vi "Main.vi"() -> ()   [LabVIEW 2019]
doc: "管道泄漏检测系统主程序"
uses:
  SSH Library/Connection Info..cluster.ctl
  SSH Library/Password..cluster.ctl
  References/PythonVersionsEnum.ctl
  <vilib>/Utility/miscctls.llb/LVForegroundBackgroundColorsTypeDef.ctl
  SSH Library/connect_password.vi
  SSH Library/connect_key.vi
  SFTP Library/connect_password.vi
  SFTP Library/connect_key.vi
  <vilib>/Utility/file.llb/Read Delimited Spreadsheet (DBL).vi
  SSH Library/LabSSH.lvlib
  SFTP Library/LabSFTP.lvlib
panel:
  out "泄漏点位置":sgl
  in  "管长":i32=100
  in  "时间间隔":string="10"
  in  "重复次数":string="3"
  in  "开始时间":string="140300"
  in  "开始日期":string="20200810"
  in  "增益":string="1"
  in  "采样率":string="6"
  out "混合信号图":T1(graph)
  in  "关闭":bool
  in  "运行":bool
  in  "选项卡控件":enum32{"系统模型", "设备参数设置", "输出显示"}(tab)=enum."设备参数设置"
  out "布尔 10":bool
  out "布尔 9":bool
  out "Multi-Segment Pipe 2":bool(c317)
  out "布尔 8":bool
  out "布尔 7":bool
  out "布尔 6":bool
  out "布尔 5":bool
  out "布尔 4":bool
  out "布尔 3":bool
  out "布尔 2":bool
  out "Multi-Segment Pipe":bool(c317)
  in  "1号设备连接信息":T2={"IP地址"="192.168.137.140", "用户名"="pi", "端口 (22)"=22}
  in  "Password 1":T3={"密码"="zjl"}
  out "isSshConnected":bool
  out "SSH响应":string
  in  "Connection Type":enum16{"Password", "Private Key"}(ring)
  in  "Expected Response":string="raspberrypi："
  in  "Password 2":T3={"密码"="raspberry"}
  in  "2号设备连接信息":T2={"IP地址"="192.168.137.224", "用户名"="pi", "端口 (22)"=22}
  in  "Password 3":T3={"密码"="raspberry"}
  in  "3号设备连接信息":T2={"IP地址"="192.168.137.224", "用户名"="pi", "端口 (22)"=22}
  out "SFTP响应":string
  out "isSftpConnected":bool
  out "Output":string
  out "运行状态":bool
  out "诊断结论":string
  in  "采样点数":string="2000"
  in  "通道号":string="0"
  out "进度条":dbl(slide) scale=0.0..1.0
  out "开始时间":dbl=18702.3337437 caption="相对秒钟" format="%_19f"
  in  "采集命令":string="cd /home/pi/leakad\nsudo ./pipedaq  0  2000  5  1"
  out "日期字符串":string="2020/5/27"
  out "时间字符串":string="13:45:51"
  # "管道泄漏监测系统"
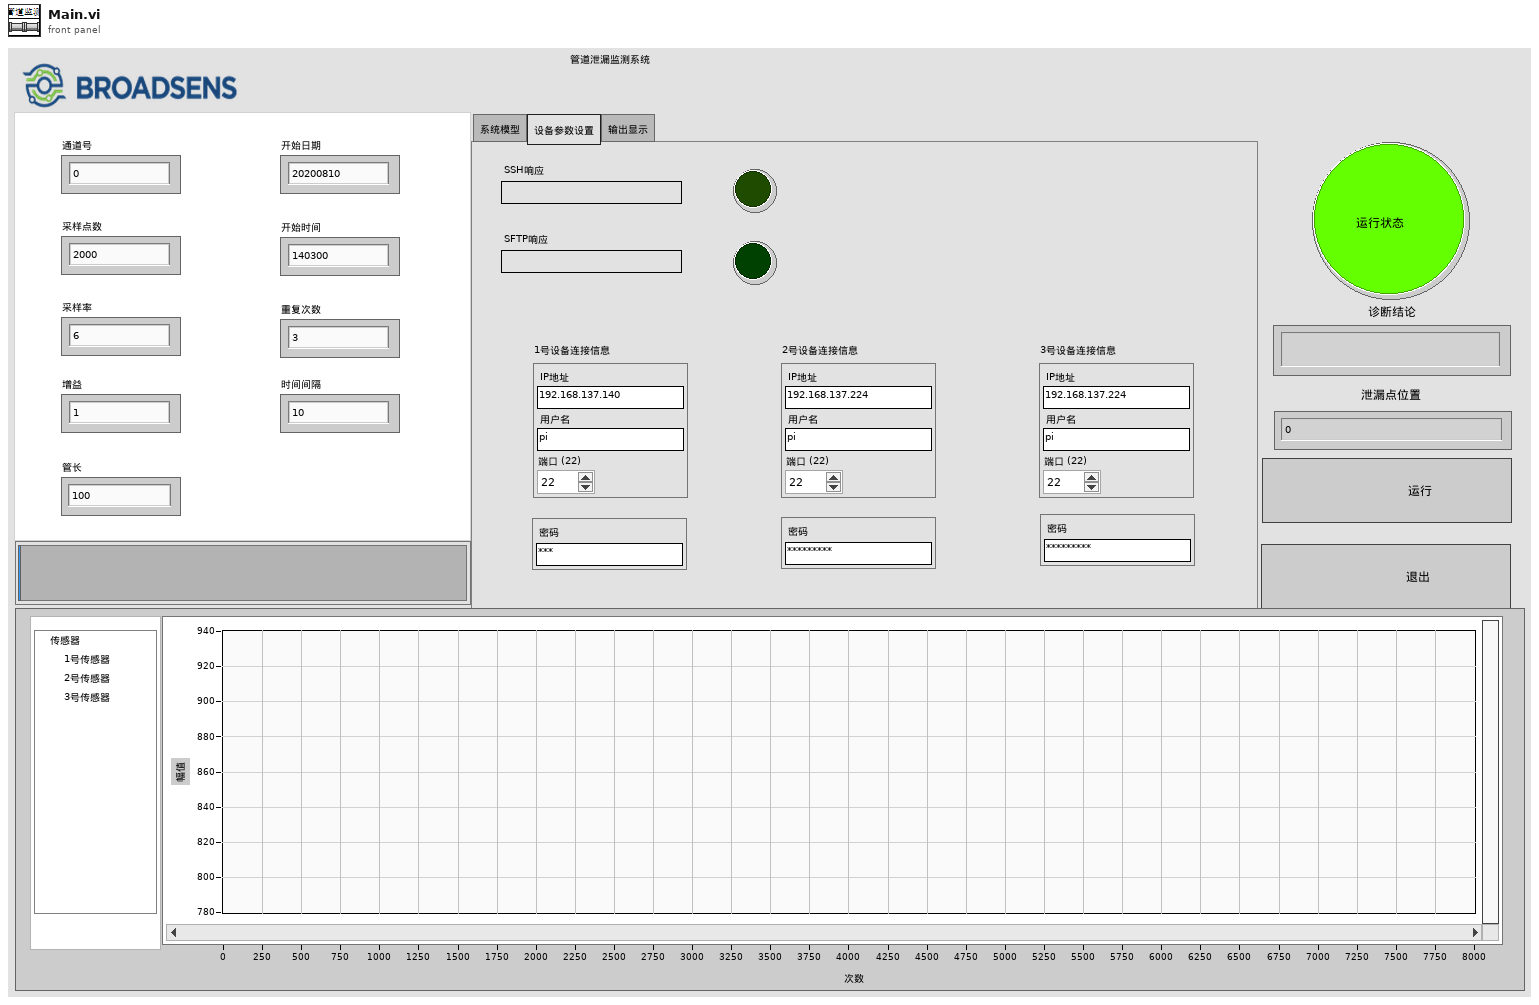
[diagram p1: front panel]
types:
  T1 = cluster{"first row":dbl[], "first row":dbl[], "first row":dbl[]}
  T2 = typedef "LabSSH.lvlib/Connection Info..cluster.ctl" = cluster{"IP地址":string, "用户名":string, "端口 (22)":i32}
  T3 = typedef "LabSSH.lvlib/Password..cluster.ctl" = cluster{"密码":string}
  T4 = enum32{"Invalid", "Standard", "Closed", "Hidden", "Minimized", "Maximized"}
  T5 = enum32{"invalid app kind", "Development System", "Run Time System", "Student Edition", "Embedded LabVIEW", "Evaluation", "Custom"}
  T6 = typedef "PythonVersionsEnum.ctl" = enum16{"2.7", "3.6"}
  T7 = typedef "LVForegroundBackgroundColorsTypeDef.ctl" = cluster{"Foreground Color":u32, "Background Color":u32}
  T8 = cluster{"Core":cluster{"Current VI Reference":refnum<vi>, "Close Panel on Exit?":bool}, "Your Boolean data":bool, "Your string data":string}
  T9 = cluster{"Current VI Reference":refnum<vi>, "Close Panel on Exit?":bool}
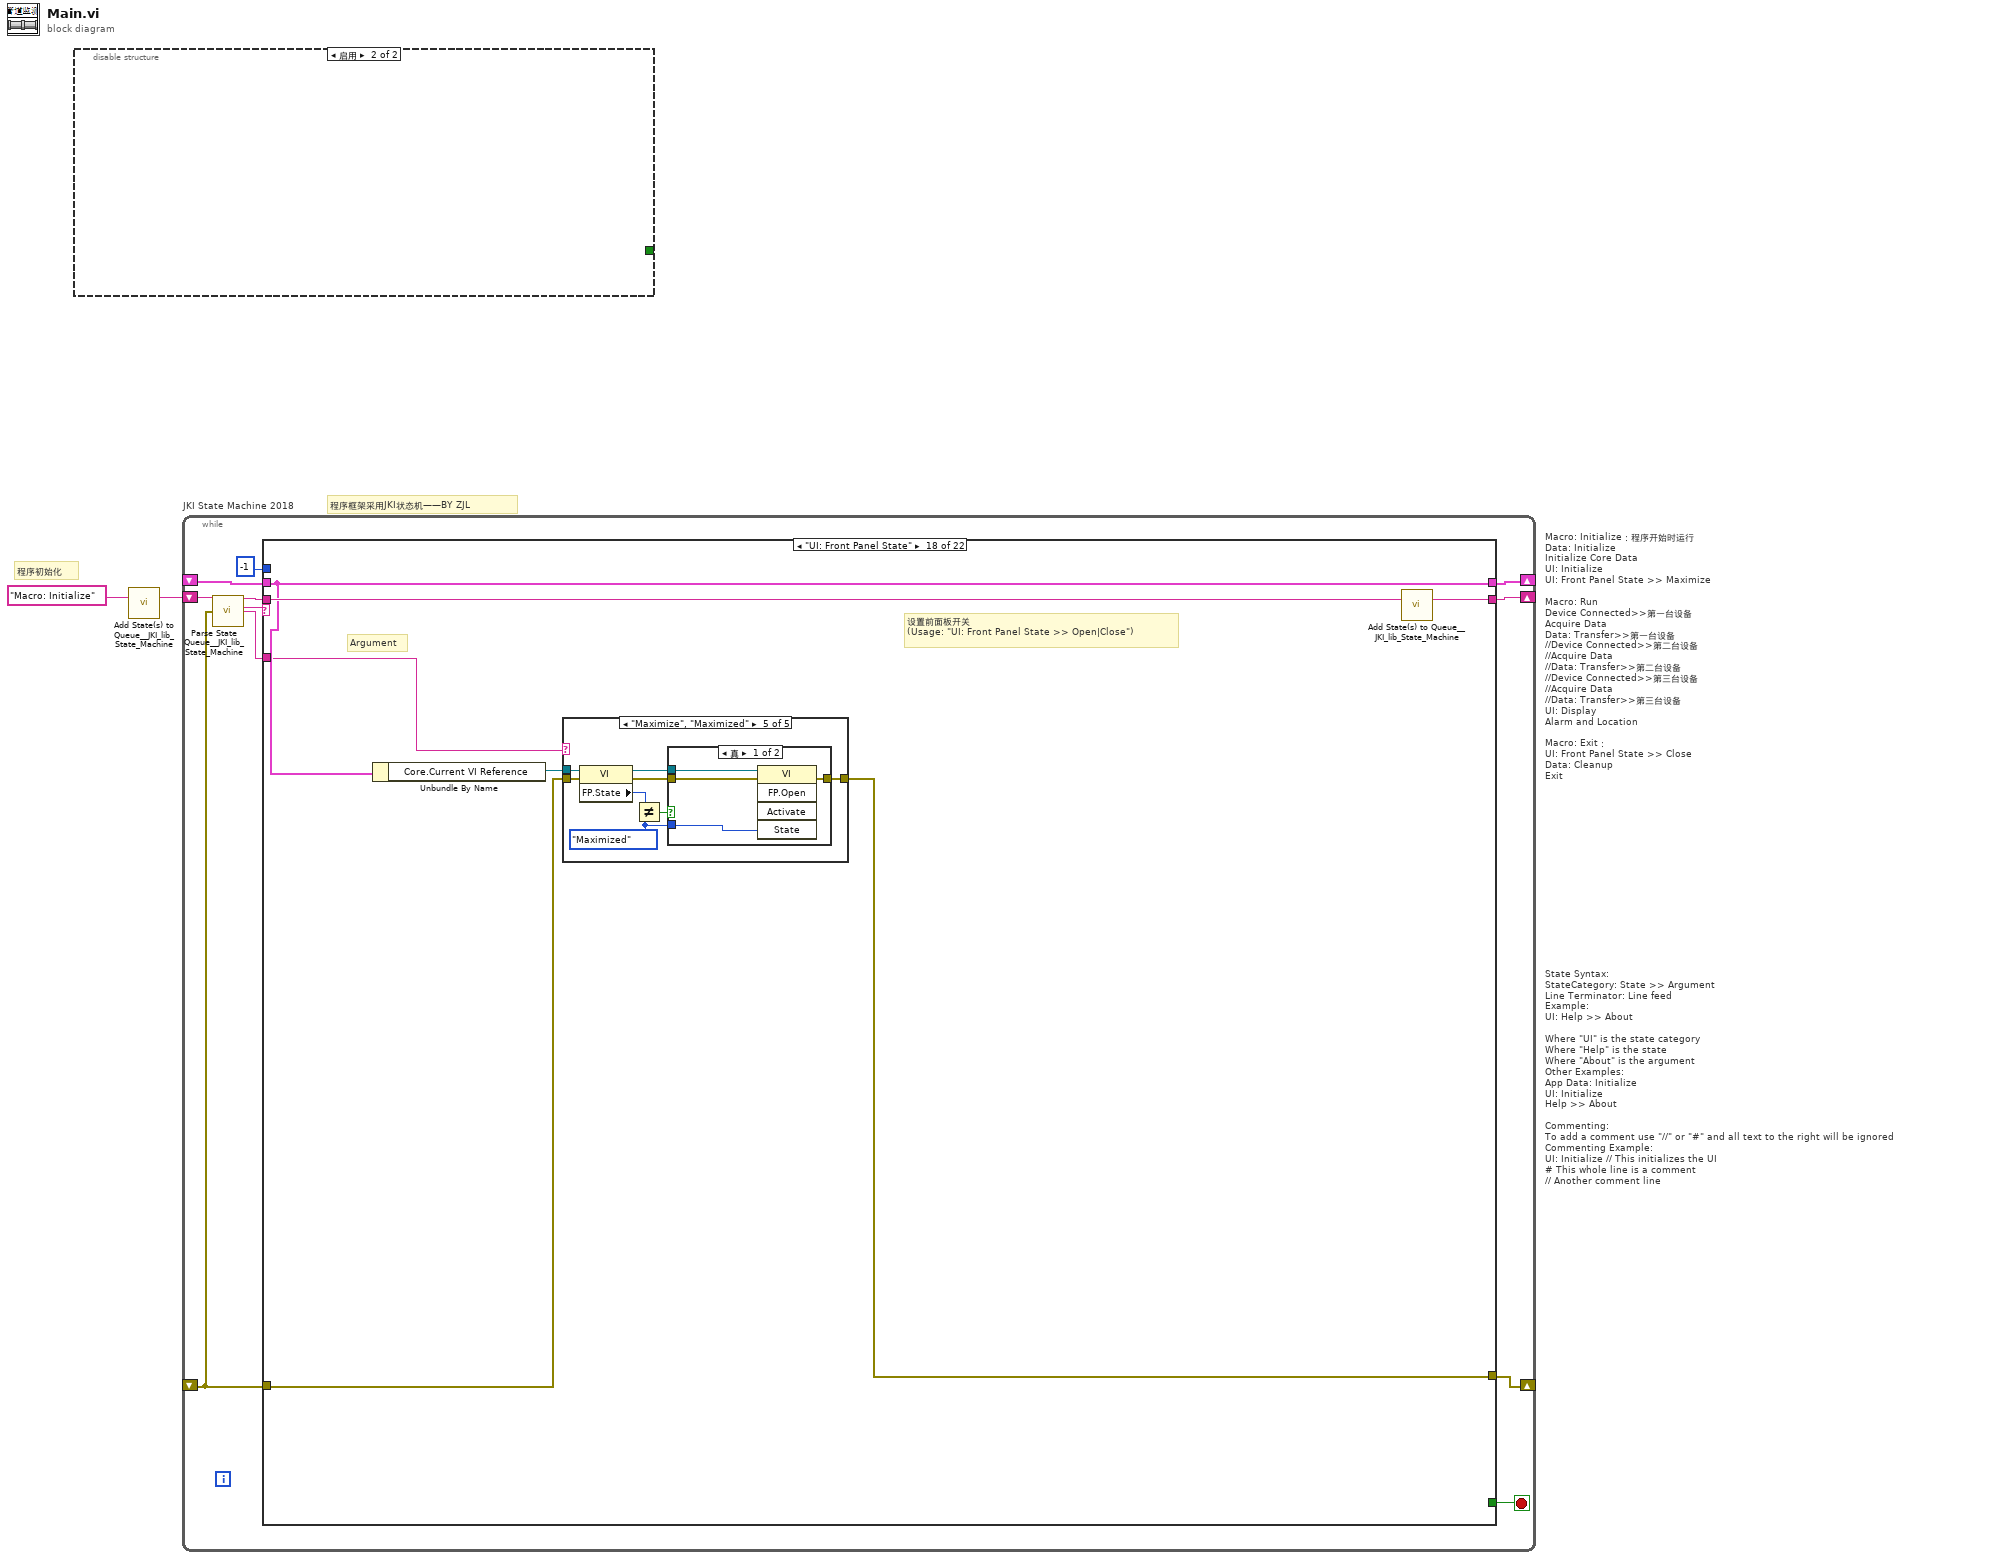
[diagram p0: block diagram]
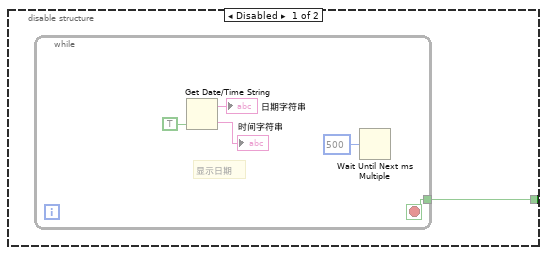
[diagram p2: hidden frame]
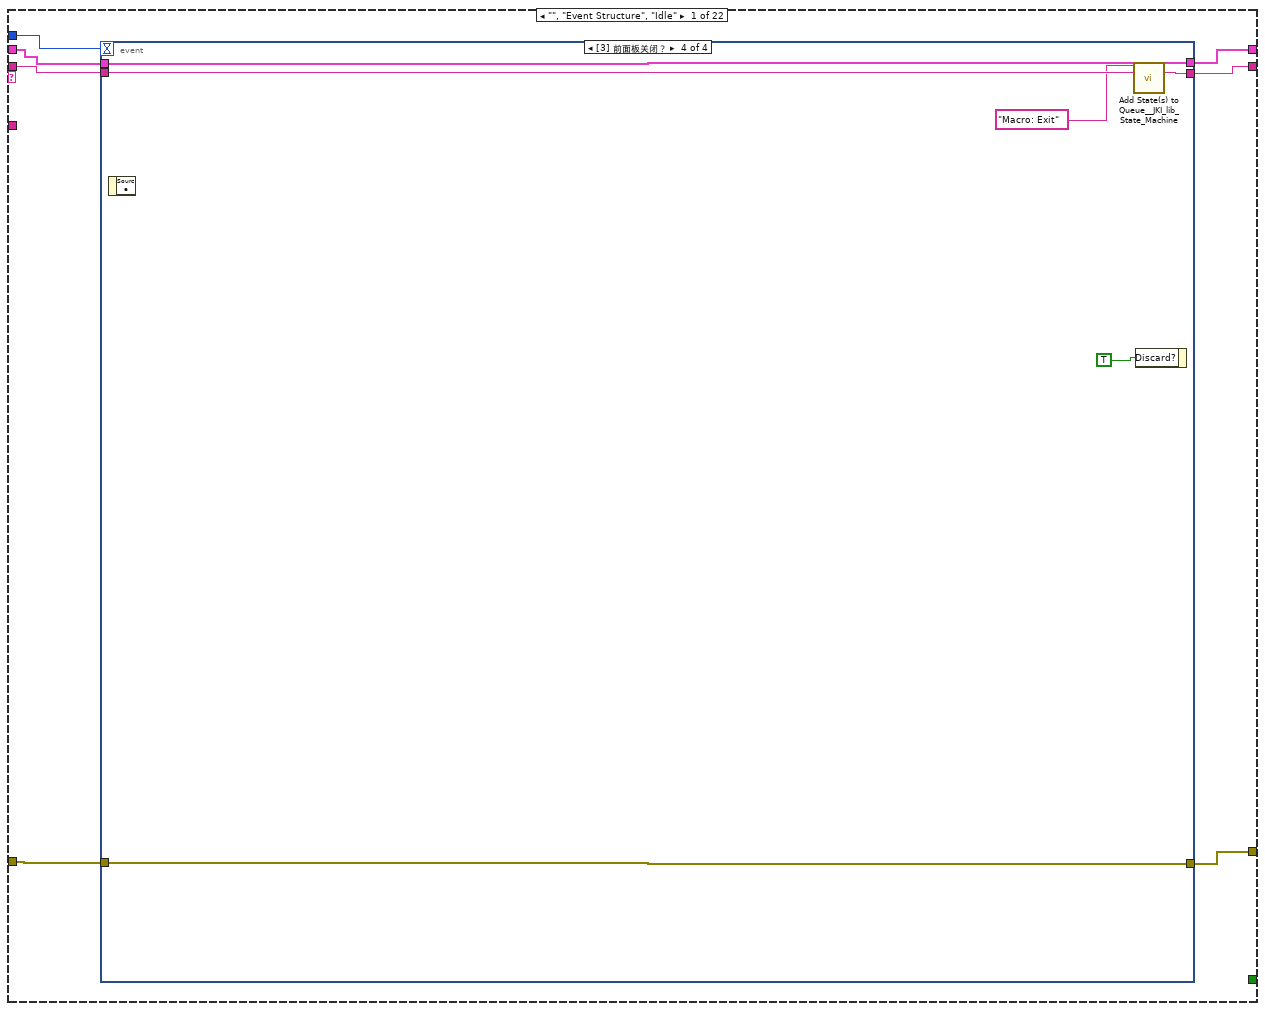
[diagram p3: hidden frame]
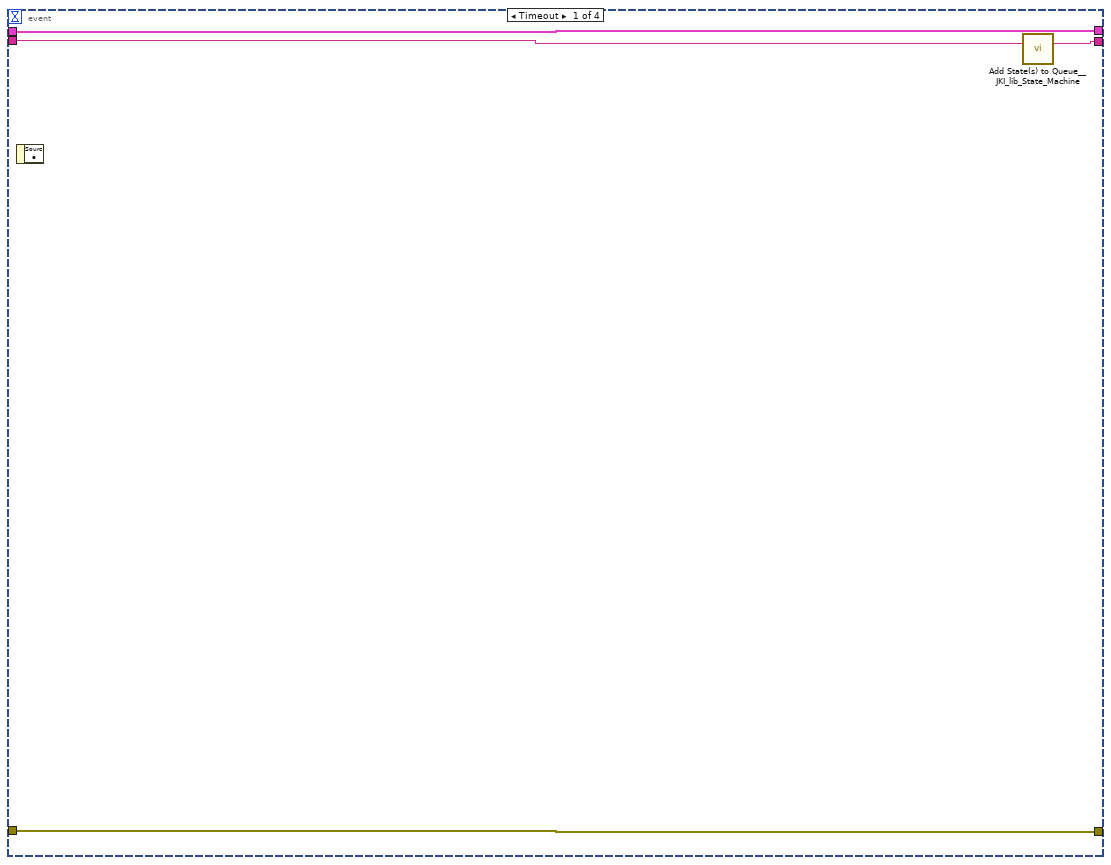
[diagram p4: hidden frame]
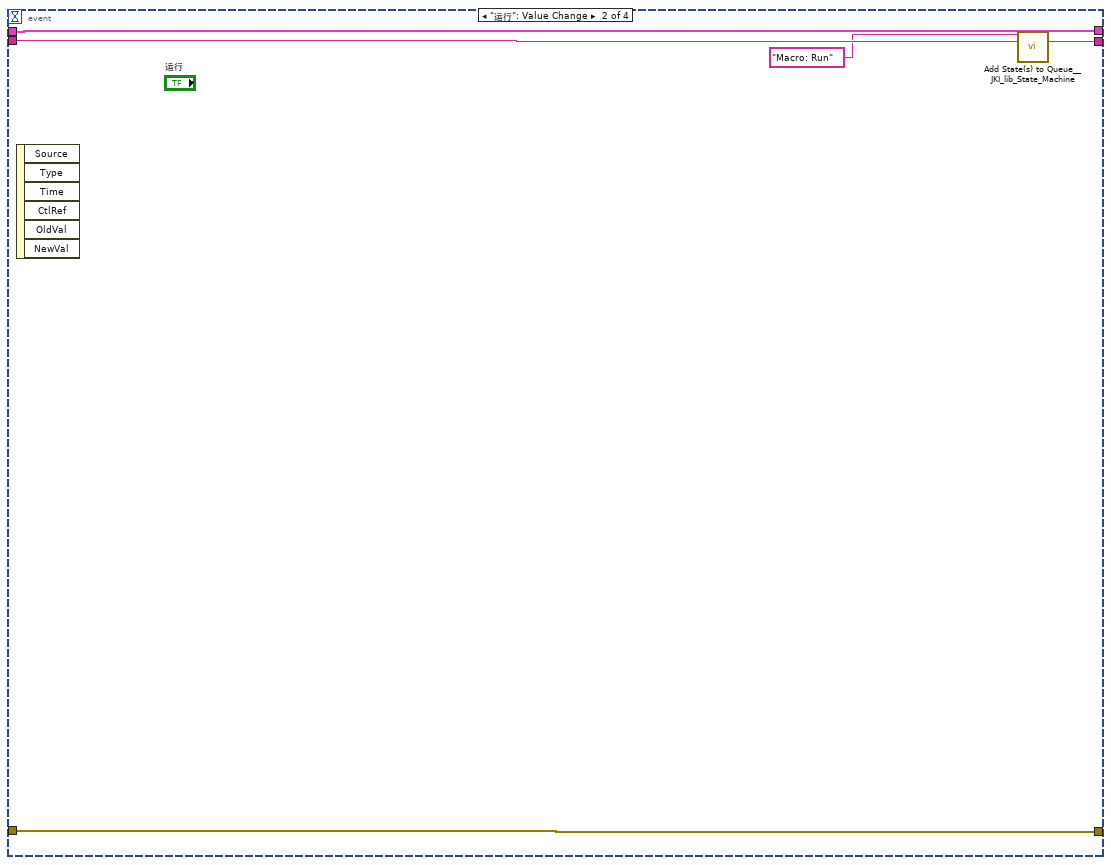
[diagram p5: hidden frame]
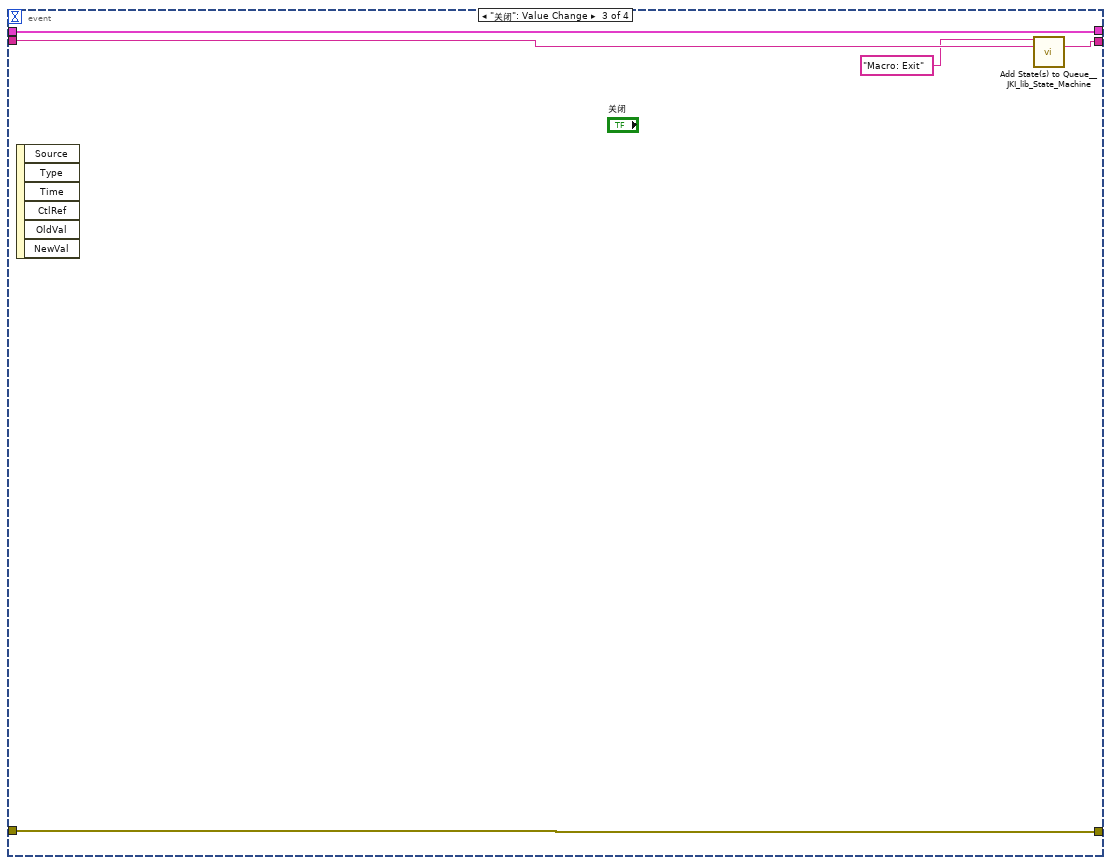
[diagram p6: hidden frame]
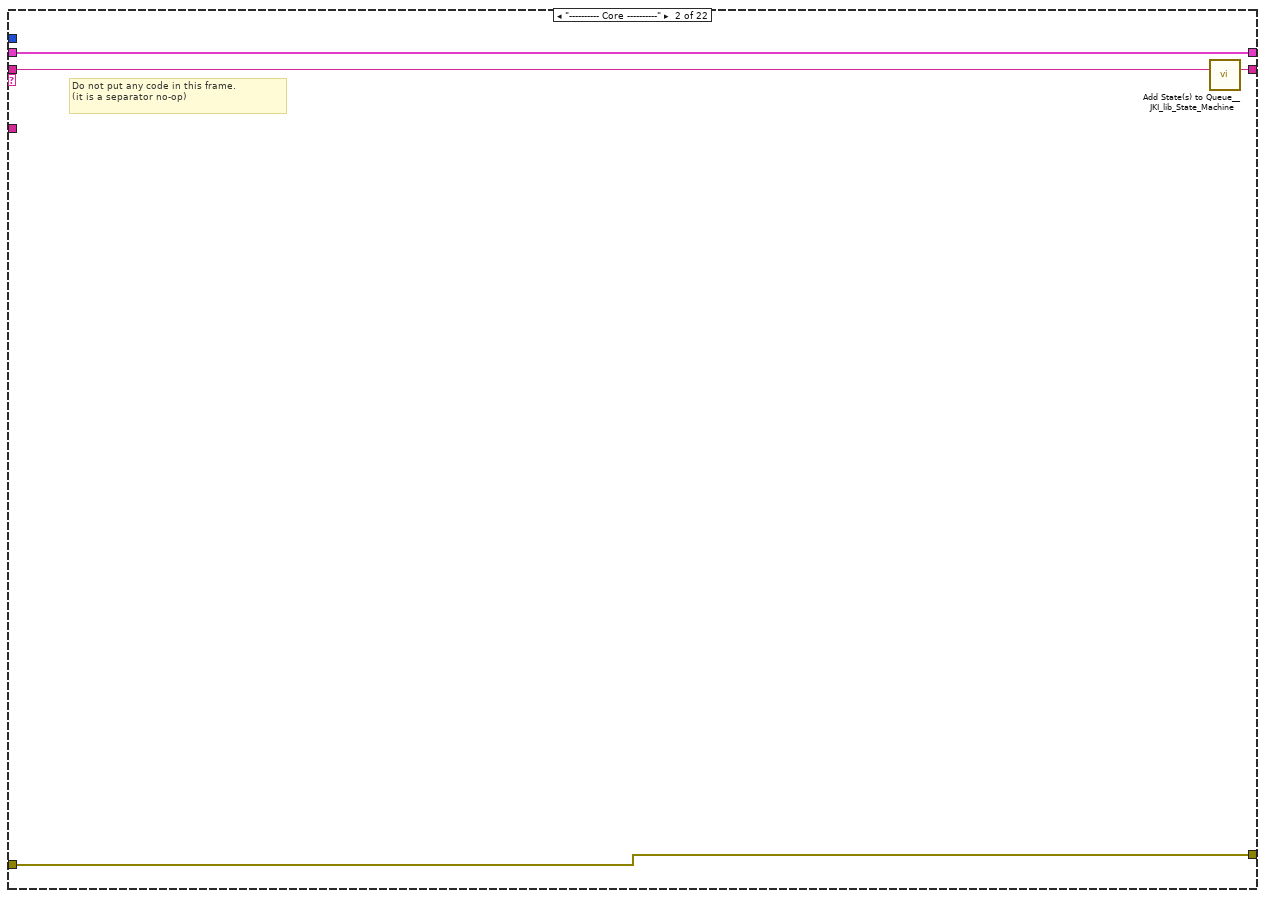
[diagram p7: hidden frame]
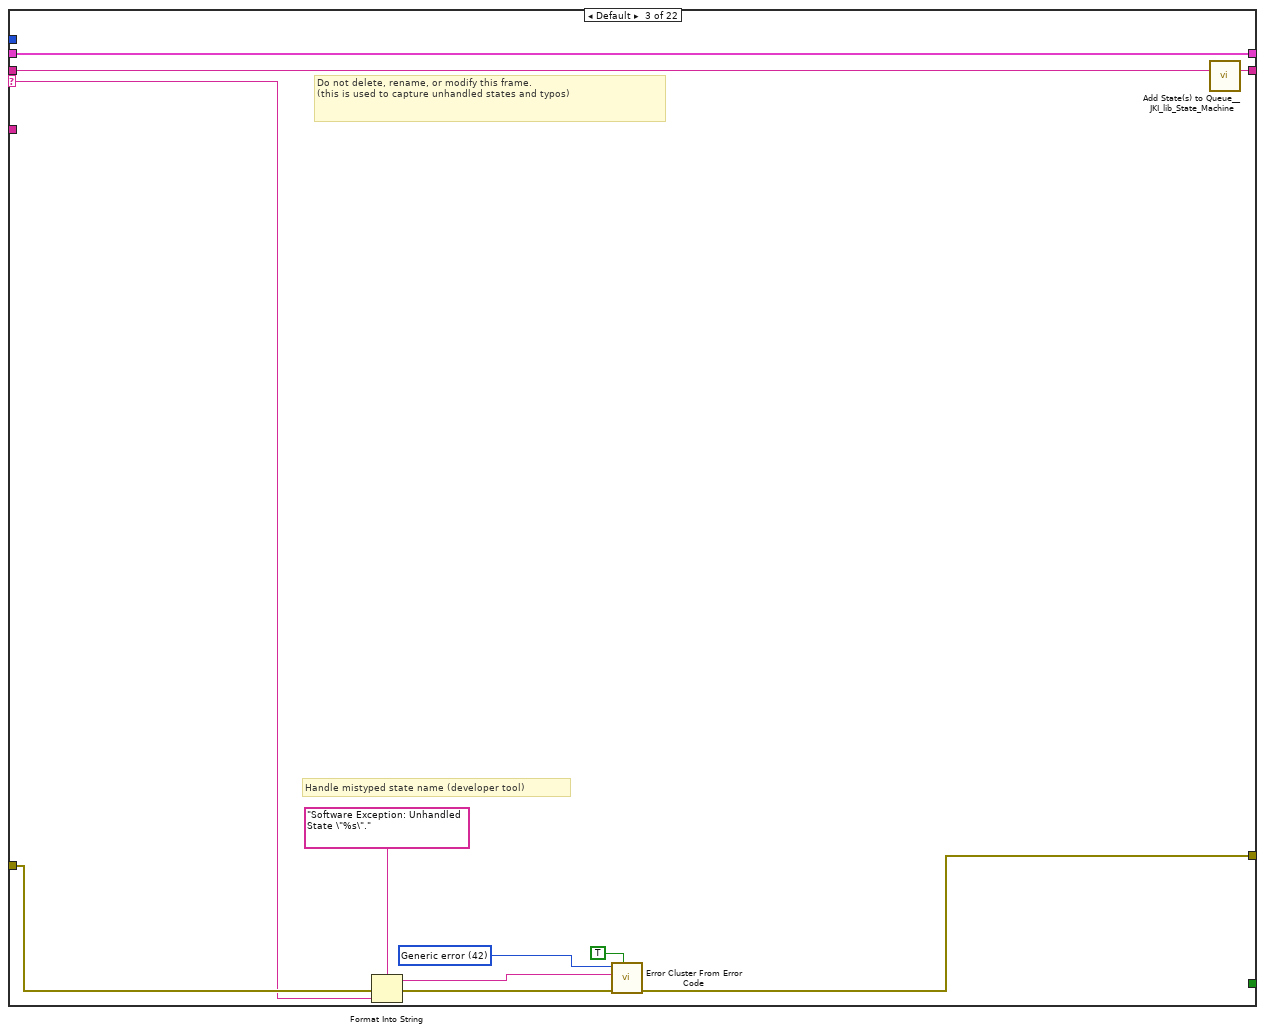
[diagram p8: hidden frame]
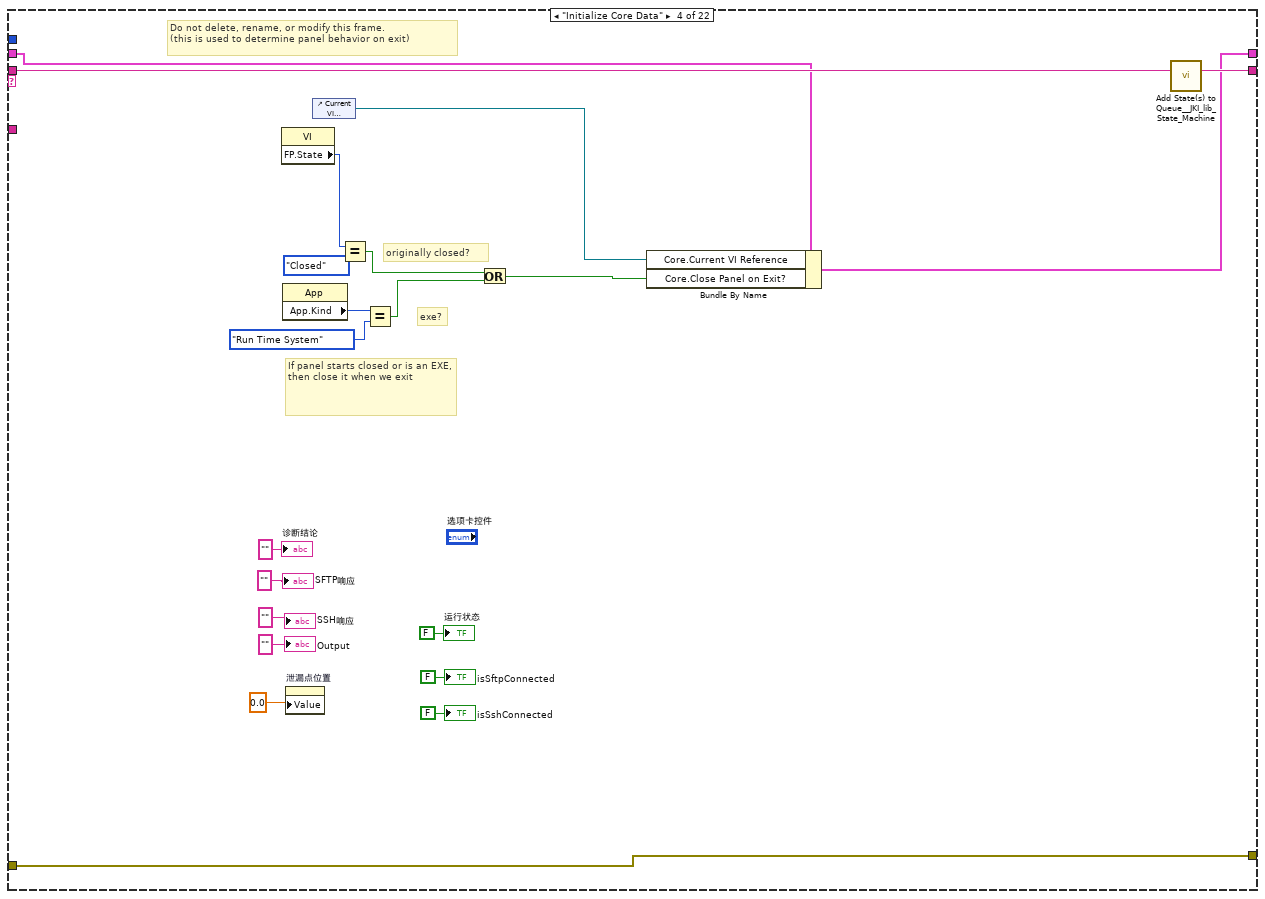
[diagram p9: hidden frame]
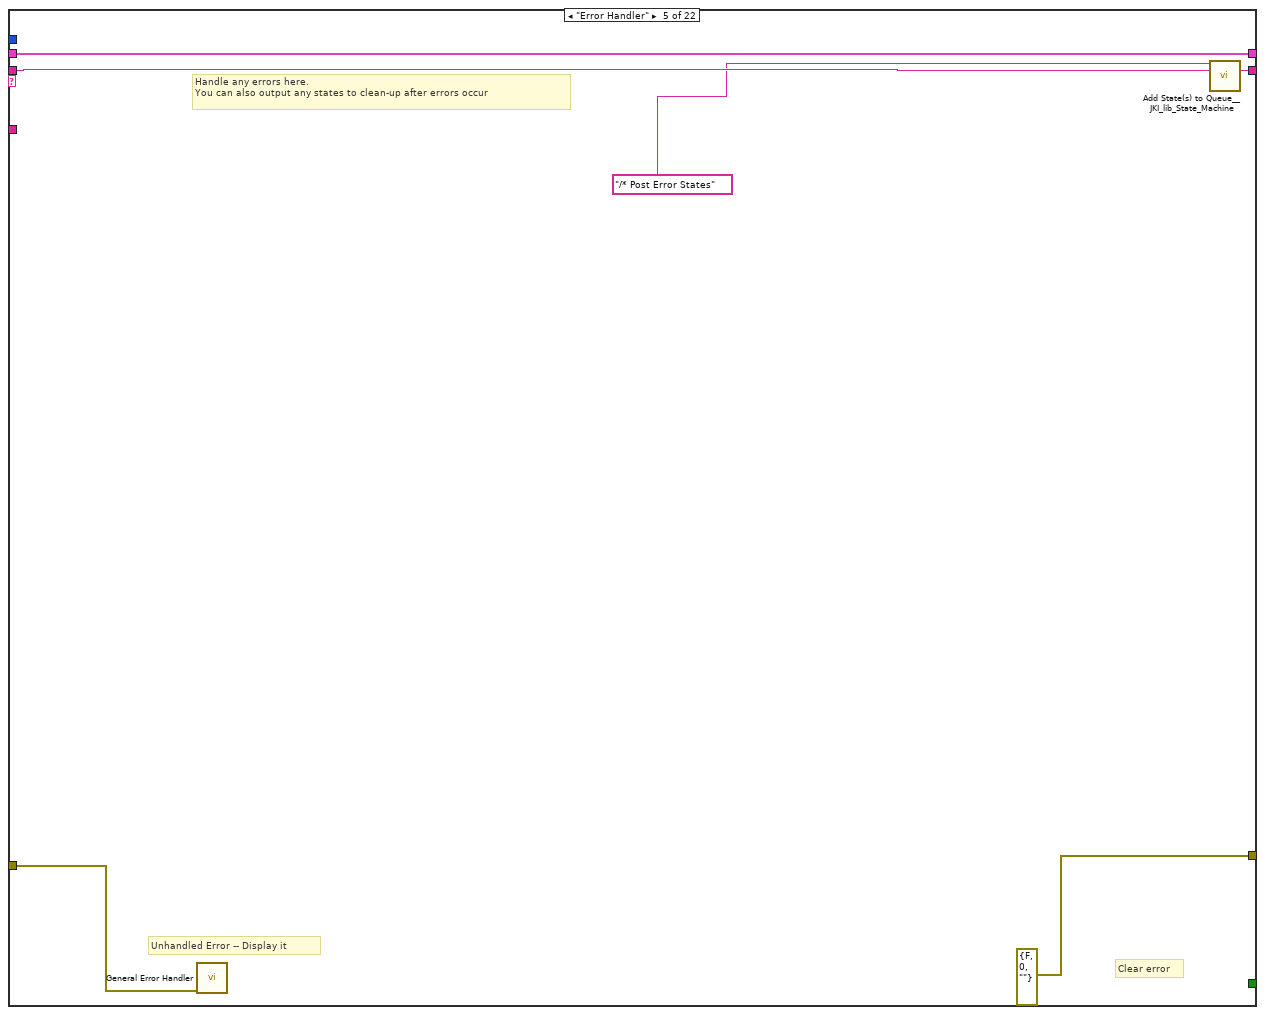
[diagram p10: hidden frame]
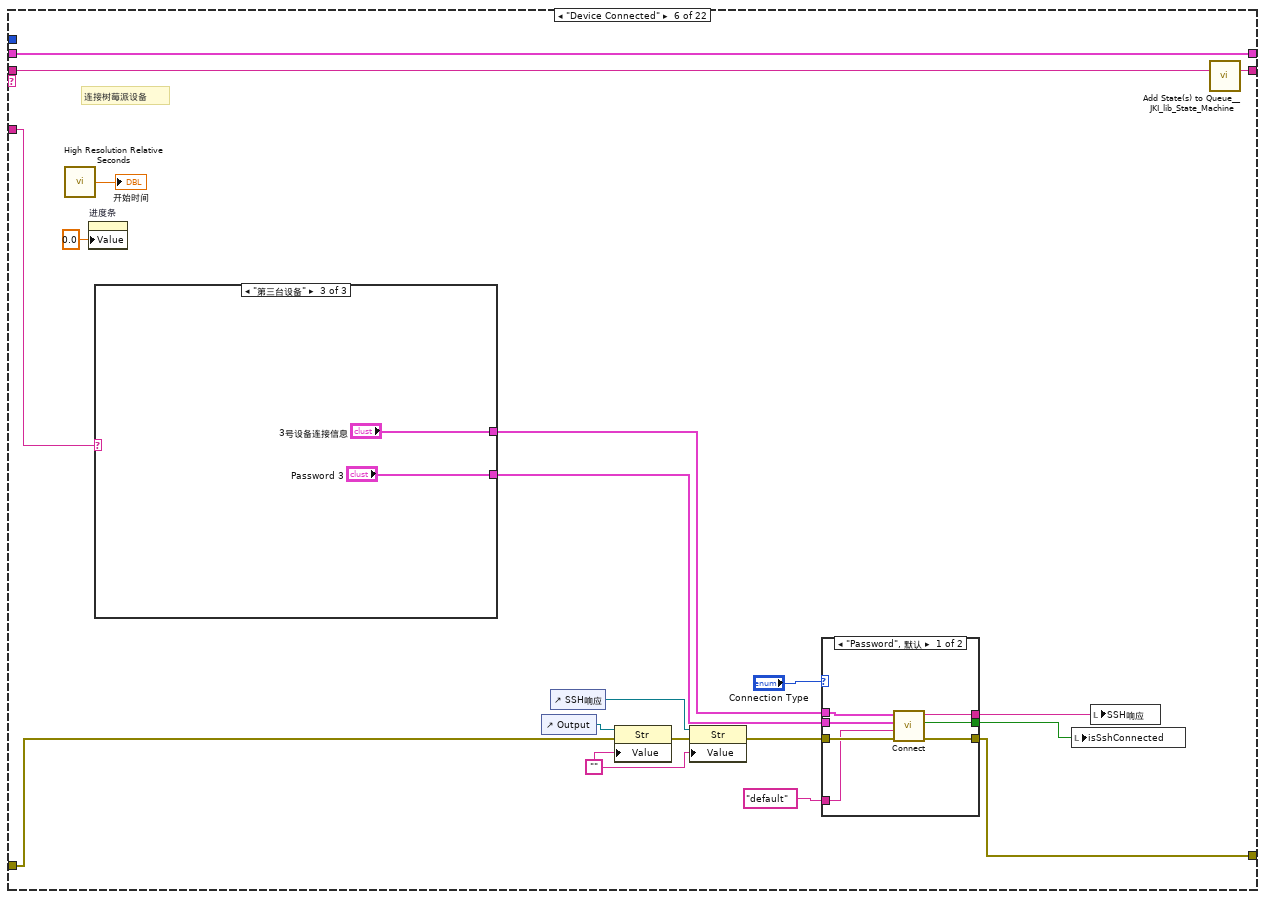
[diagram p11: hidden frame]
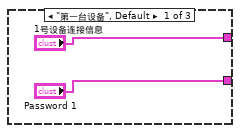
[diagram p12: hidden frame]
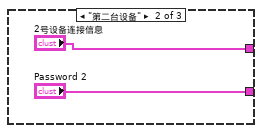
[diagram p13: hidden frame]
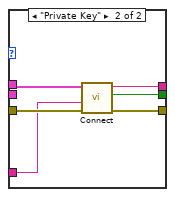
[diagram p14: hidden frame]
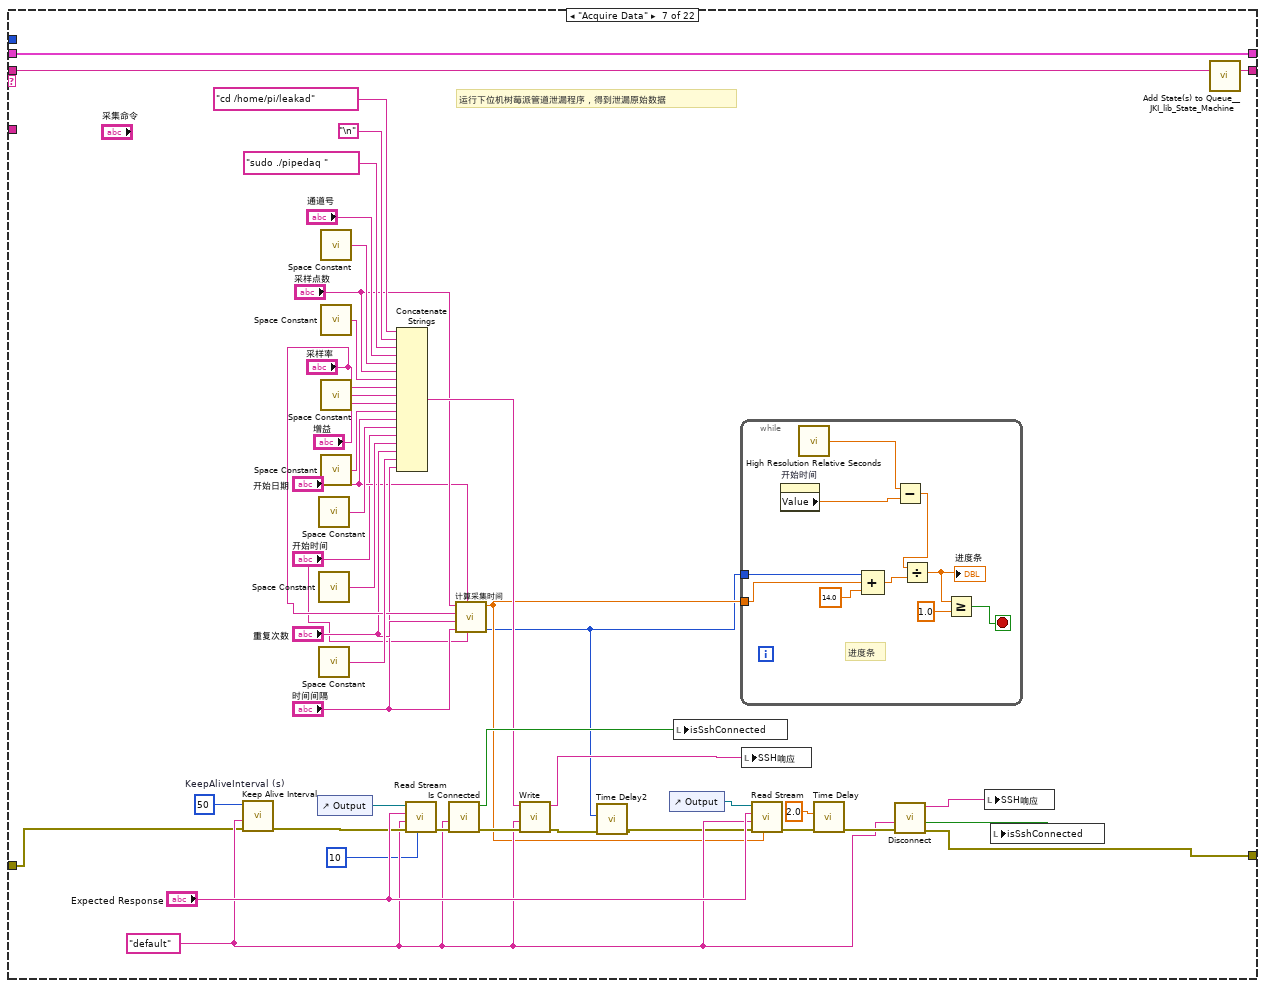
[diagram p15: hidden frame]
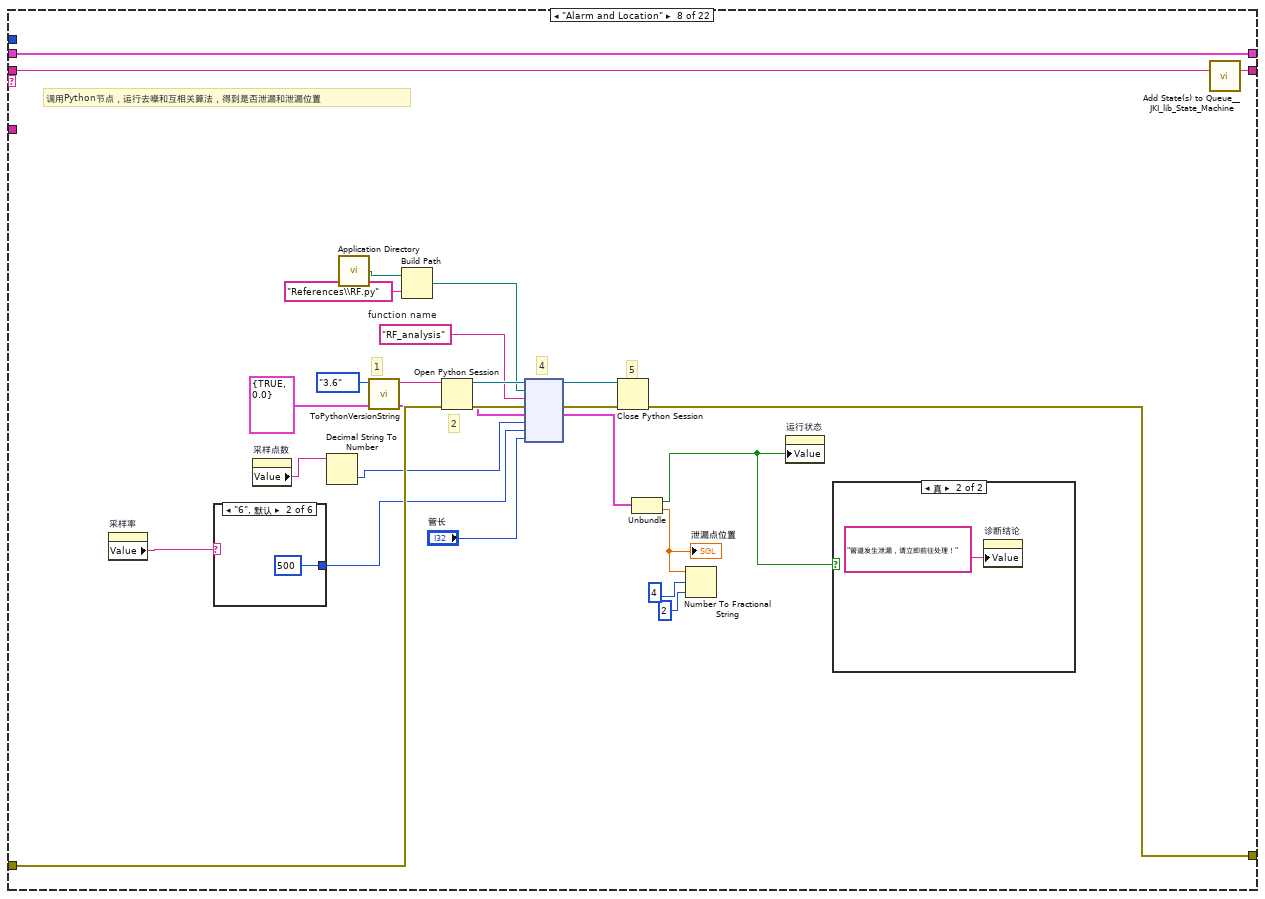
[diagram p16: hidden frame]
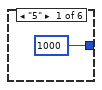
[diagram p17: hidden frame]
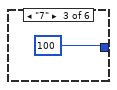
[diagram p18: hidden frame]
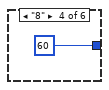
[diagram p19: hidden frame]
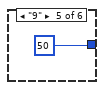
[diagram p20: hidden frame]
diagram:
  # "State Syntax:\nStateCategory: State >> Argument\nLine Terminator: Line feed\nExample:\nUI: Help >> About\n\nWhere \"UI\" is the state category\nWhere \"Help\" is the state\nWhere \"About\" is the argument\nOther Examples:\nApp Data: Initialize\nUI: Initialize\nHelp >> About\n\nCommenting:\nTo add a comment use \"//\" or \"#\" and all text to the right will be ignored\nCommenting Example:\nUI: Initialize // This initializes the UI\n# This whole line is a comment\n// Another comment line"
  # "程序初始化"
  # "程序框架采用JKI状态机——BY ZJL"
  # "Macro: Initialize：程序开始时运行\nData: Initialize\nInitialize Core Data\nUI: Initialize\nUI: Front Panel State >> Maximize\n\nMacro: Run\nDevice Connected>>第一台设备\nAcquire Data\nData: Transfer>>第一台设备\n//Device Connected>>第二台设备\n//Acquire Data\n//Data: Transfer>>第二台设备\n//Device Connected>>第三台设备\n//Acquire Data\n//Data: Transfer>>第三台设备\nUI: Display\nAlarm and Location\n\nMacro: Exit：\nUI: Front Panel State >> Close\nData: Cleanup \nExit"
  n1 = disable-structure shown="启用" {
    disable-tunnel: _ -> [w3 _]
    frame Disabled {
      n2 = while {
        tunnel: w3 -> [w4]
        stop <- w4 stop-if-true
        # "显示日期"
        n3 = Get Date/Time String(want seconds? (F)=TRUE ("需要秒？(F)")) -> (date string=→"日期字符串":string, time string=→"时间字符串":string)  [unwired: 2 in]
        n4 = Wait Until Next ms Multiple(millisecond multiple=u32 500 ("毫秒倍数")) -> ()  [unwired: 1 out]
      }
    }
    frame Enabled {
    }
  }
  n5 = call <vilib>:"Add State(s) to Queue__JKI_lib_State_Machine.vi"("State(s) in (\"\")"="Macro: Initialize") -> ("States Out"=w2:string)  [unwired: 14 in]
  n6 = while "JKI State Machine 2018" {
    shift-right: [w13] -> _
    shift-left: _ -> [w12]
    shift-right: [w15] -> _
    shift-left: _ -> [w10]
    shift-right: [w14] -> _
    shift-left: w2 -> [w16]
    stop <- w9 stop-if-true
    n7 = call <vilib>:"Parse State Queue__JKI_lib_State_Machine.vi"("State Queue"=w16, "Error In (no error)"=w10) -> ("Remaining States"=w18:string, "Current State"=w19:string, "Arguments"=w17:string)  [unwired: 11 in]
    n8 = case "条件结构" shown="\"UI: Front Panel State\"" w19 {
      selector: w19 -> [_ _ w51 _ _ _ _ _ _ _ _ _ _ _ _ _ _ _ _ _ _ _]
      tunnel: w18 -> [w26 w50 w55 w82 w88 w107 w170 w206 w219 w223 w230 w260 w290 w294 w300 w346 w352 w363 w432 w437 w442 w452]
      tunnel: w17 -> [_ _ _ _ _ w93 _ _ _ _ _ w246 _ _ _ _ w347 w357 _ _ _ _]
      tunnel: w12 -> [w24 w47 w53 w75 w85 w105 w168 w204 w217 w220 _ w258 w285 w291 w298 w343 w350 w359 w429 w434 w439 w449]
      tunnel: [w23 w48 w57 w79 errorcluster {"status"=FALSE, "code"=0, "source"=""} ("error out") w94 w138 w202 w216 w221 w227 w240 w286 w292 w296 w344 w348 w360 w430 w435 w440 w450] -> w15
      tunnel: w10 -> [w22 w48 w56 w79 w84 w95 w158 w203 w216 w221 w227 w250 w287 w292 w295 w344 w349 w361 w430 w435 w440 w450]
      tunnel: [w25 w49 w54 w81 w87 w106 w169 w205 w218 w222 w229 w259 w289 w293 w299 w345 w351 w362 w431 w436 w441 w451] -> w14
      tunnel: [_ _ _ _ _ _ _ _ TRUE _ _ _ _ _ _ _ _ _ _ _ _ _] -> w9
      tunnel: [w21 w47 w53 w80 w85 w105 w168 w204 w217 w220 w228 w258 w285 w291 w298 w343 w350 w359 w429 w434 w439 w449] -> w13
      tunnel: -1 -> [w20 _ _ _ _ _ _ _ _ _ _ _ _ _ _ _ _ _ _ _ _ _]
      frame "", "Event Structure", "Idle" {
        n9 = event shown="[3] 前面板关闭？" {
          selector: _ -> [_ _ _ _]
          dyn-events: _ -> [_ _ _ _]
          timeout: w20 -> [_ _ _ _]
          tunnel: w26 -> [w30 w33 w40 w46]
          tunnel: [w29 w34 w39 w45] -> w25
          tunnel: w24 -> [w27 w35 w37 w43]
          tunnel: [w28 w31 w38 w44] -> w23
          tunnel: w22 -> [w28 w31 w38 w44]
          tunnel: [w27 w35 w37 w43] -> w21
          event Timeout {
            n10 = event-data() -> ()  [unwired: 1 in, 1 out]
            n11 = call <vilib>:"Add State(s) to Queue__JKI_lib_State_Machine.vi"("State(s) in (\"\")"=w30) -> ("States Out"=w29:string)  [unwired: 14 in]
          }
          event "运行": Value Change {
            n12 = event-data() -> ()  [unwired: 1 in, 6 out]
            n13 = call <vilib>:"Add State(s) to Queue__JKI_lib_State_Machine.vi"("State(s) in Front (\"\")"="Macro: Run" ("State(s) in Front (\"\")"), "State(s) in (\"\")"=w33) -> ("States Out"=w34:string)  [unwired: 13 in]
          }
          event "关闭": Value Change {
            n14 = event-data() -> ()  [unwired: 1 in, 6 out]
            n15 = call <vilib>:"Add State(s) to Queue__JKI_lib_State_Machine.vi"("State(s) in Front (\"\")"="Macro: Exit", "State(s) in (\"\")"=w40) -> ("States Out"=w39:string)  [unwired: 13 in]
          }
          event Panel Close? {
            n16 = event-data() -> ()  [unwired: 1 in, 1 out]
            n17 = call <vilib>:"Add State(s) to Queue__JKI_lib_State_Machine.vi"("State(s) in Front (\"\")"="Macro: Exit", "State(s) in (\"\")"=w46) -> ("States Out"=w45:string)  [unwired: 13 in]
            n18 = event-data("Discard?"=TRUE) -> ()  [unwired: 1 in, 1 out]
          }
        }
      }
      frame "---------- Core ----------" {
        # "Do not put any code in this frame.\n(it is a separator no-op)"
        n19 = call <vilib>:"Add State(s) to Queue__JKI_lib_State_Machine.vi"("State(s) in (\"\")"=w50) -> ("States Out"=w49:string)  [unwired: 14 in]
      }
      frame Default {
        w60 = 42 items=["No error", "Argument error", "Memory is full", "Out of zone", "End of file", "File already open", "Generic file I/O error", "File not found", "File permission error", "Disk is full", "Duplicate path", "Too many files open", "System feature not enabled", "Resource file not found", "Cannot add resource", "Resource not found", "Image not found", "Image memory error", "Pen does not exist", "Config type invalid", "Config token not found", "Config parse error", "Config memory error", "Bad external code format", "Bad external code offset", "External code not present", "Null window", "Destroy window error", "Null menu", "Print aborted", "Bad print record", "Print driver error", "Windows error during printing", "Memory error during printing", "Print dialog error", "Generic print error", "Invalid device refnum", "Device not found", "Device parameter error", "Device unit error", "Cannot open device", "Device call aborted", "Generic error", "Cancelled by user", "Object ID too low", "Object ID too high", "Object not in heap", "Unknown heap", "Unknown object (invalid DefProc)", "Unknown object (DefProc not in table)", "Message out of range", "Invalid (null) method", "Unknown message", "Manager call not supported", "Bad address", "Network operation in progress", "Network operation timed out", "Connection is busy", "Network attribute not supported", "Network error", "Address in use", "System out of memory", "Connection aborted", "Connection refused", "Not connected", "Already connected", "Connection closed", "Initialization error (interapplication manager)", "Bad occurrence", "Wait on unbound occurrence handler", "Occurrence queue overflow", "Datalog type conflict", "Unused", "Unrecognized type (interapplication manager)", "Memory corrupt", "Failed to make temporary DLL", "Old CIN version", "Drag socket not found", "Failed to load drop-object", "Failed to register OLE object", "Failed to release OLE object", "Format specifier type mismatch", "Unknown format specifier", "Too few format specifiers", "Too many format specifiers", "Scan failed", "Newer CIN version", "Error converting to variant", "Runtime menu error", "Password tampered", "Variant attribute not found", "Incompatible variant data type", "Event data is not available", "Event Store is not present", "Occurrence is not found", "Event Queue is not created", "Event info is not available", "Refnum passed is NULL", "Error retrieving Class GUID", "Error retrieving CoClass GUID", "Error retrieving TypeLib GUID.", "Bad built application magic bytes.", "Specific driver is different from the specific driver associated with the Logical Name.", "There is no session opened to the class driver.", "Max Error", "MAX - Error with config objects", "MAX - Error loading configuration", "MAX - Group not supported"]
        # "Do not delete, rename, or modify this frame.\n(this is used to capture unhandled states and typos)"
        # "Handle mistyped state name (developer tool)"
        n20 = Format Into String(format string="Software Exception: Unhandled State \"%s\"." ("message"), error in=w56, w51) -> (resulting string=w59:string, error out=w58:errorcluster)  [unwired: 1 in]
        n21 = call <vilib>:"Error Cluster From Error Code.vi"("show call chain? (False)"=TRUE, "error in (no error)"=w58, "error message (\"\")"=w59, "error code (0)"=w60) -> ("error out"=w57:errorcluster)  [unwired: 5 in]
        n22 = call <vilib>:"Add State(s) to Queue__JKI_lib_State_Machine.vi"("State(s) in (\"\")"=w55) -> ("States Out"=w54:string)  [unwired: 14 in]
      }
      frame "Initialize Core Data" {
        # "Do not delete, rename, or modify this frame.\n(this is used to determine panel behavior on exit)"
        # "originally closed?"
        # "exe?"
        # "If panel starts closed or is an EXE, then close it when we exit"
        n23 = property class="VI"() -> ("FP.State"=w72:T4)  [unwired: 2 in, 2 out]
        n24 = property class="App"() -> ("App.Kind"=w78:T5)  [unwired: 2 in, 2 out]
        n25 = property on="泄漏点位置" class="DigNum (严格)"("Value"=sgl 0.0) -> ()  [unwired: 2 in, 2 out]
        n26 = control-ref of="Current VI Reference"() -> (w73:refnum<vi>)
        n27 = Equal?(x=w72, y=T4."Closed" ("Front Panel Window:State")) -> (x = y?=w70:bool)
        n28 = Equal?(x=w78, y=T5."Run Time System" ("Application:Kind")) -> (x = y?=w76:bool)
        n29 = Or(x=w70, y=w76) -> (x .or. y?=w74:bool)
        n30 = Bundle By Name(cluster=w75, "Core.Current VI Reference"=w73, "Core.Close Panel on Exit?"=w74) -> (w80:T8)
        n31 = call <vilib>:"Add State(s) to Queue__JKI_lib_State_Machine.vi"("State(s) in (\"\")"=w82) -> ("States Out"=w81:string)  [unwired: 14 in]
        "诊断结论" <- "" ("诊断结论")
        "运行状态" <- FALSE ("诊断结果")
        "isSftpConnected" <- FALSE ("isSftpConnected")
        "SFTP响应" <- "" ("SFTP响应")
        "Output" <- "" ("Output")
        "isSshConnected" <- FALSE ("isSshConnected")
        "SSH响应" <- "" ("SSH响应")
      }
      frame "Error Handler" {
        # "Unhandled Error -- Display it"
        # "Handle any errors here.\nYou can also output any states to clean-up after errors occur"
        # "Clear error"
        n32 = call <vilib>:"General Error Handler.vi"("error in (no error)"=w84) -> ()  [unwired: 10 in, 5 out]
        n33 = call <vilib>:"Add State(s) to Queue__JKI_lib_State_Machine.vi"("State(s) in Front (\"\")"="/* Post Error States", "State(s) in (\"\")"=w88) -> ("States Out"=w87:string)  [unwired: 13 in]
      }
      frame "Device Connected" {
        w98 = ""
        # "连接树莓派设备"
        n34 = call <vilib>:"High Resolution Relative Seconds.vi"() -> ("relative seconds"=→"开始时间":dbl)
        n35 = property on="进度条" class="Slide (严格)"("Value"=0.0 ("进度条")) -> ()  [unwired: 2 in, 2 out]
        n36 = case shown="\"第三台设备\"" w93 {
          tunnel: ["1号设备连接信息" "2号设备连接信息" "3号设备连接信息"] -> w92
          tunnel: ["Password 1" "Password 2" "Password 3"] -> w91
          frame "第一台设备", Default {
          }
          frame "第二台设备" {
          }
          frame "第三台设备" {
          }
        }
        n37 = control-ref of="Output"() -> (w101:refnum<vi>)
        n38 = control-ref of="SSH响应"() -> (w99:refnum<vi>)
        n39 = property class="Str"(reference=w101, error in=w95, "Value"=w98) -> (error out=w102:errorcluster)  [unwired: 1 out]
        n40 = property class="Str"(reference=w99, error in=w102, "Value"=w98) -> (error out=w100:errorcluster)  [unwired: 1 out]
        n41 = case shown="\"Password\", 默认" "Connection Type" {
          tunnel: [w120 w125] -> w94
          tunnel: w91 -> [w119 _]
          tunnel: [w118 w124] -> w104
          tunnel: [w117 w123] -> w103
          tunnel: w100 -> [w116 w126]
          tunnel: "default" ("Connection Name") -> [w115 w122]
          tunnel: w92 -> [w114 w121]
          frame "Password", Default {
            n42 = call-poly "Connect.vi"("error in (no error)"=w116, "Connection Name"=w115, "Password"=w119, "Connection Info."=w114) -> ("error out"=w120:errorcluster, "isSshConnected"=w118:bool, "Return String"=w117:string)  [unwired: 5 in]
          }
          frame "Private Key" {
            n43 = call-poly "Connect.vi"("error in (no error)"=w126, "Connection Name"=w122, "Connection Info."=w121) -> ("error out"=w125:errorcluster, "isSshConnected"=w124:bool, "Return String"=w123:string)  [unwired: 6 in]
          }
        }
        n44 = local write "isSshConnected"(w104) -> ()
        n45 = local write "SSH响应"(w103) -> ()
        n46 = call <vilib>:"Add State(s) to Queue__JKI_lib_State_Machine.vi"("State(s) in (\"\")"=w107) -> ("States Out"=w106:string)  [unwired: 14 in]
      }
      frame "Acquire Data" {
        w159 = "default" ("Connection Name")
        w160 = 50  # KeepAliveInterval (s)
        # "运行下位机树莓派管道泄漏程序，得到泄漏原始数据"
        n47 = call "Keep Alive Interval.vi"("error in (no error)"=w158, "Connection Name"=w159, "KeepAliveInterval (s)"=w160) -> ("error out"=w161:errorcluster)  [unwired: 8 in]
        n48 = control-ref of="Output"() -> (w157:refnum<vi>)
        n49 = call <vilib>:"Space Constant.vi"() -> ("String"=w142:string)
        n50 = call <vilib>:"Space Constant.vi"() -> ("String"=w141:string)
        n51 = call <vilib>:"Space Constant.vi"() -> ("String"=w140:string)
        n52 = call <vilib>:"Space Constant.vi"() -> ("String"=w147:string)
        n53 = call <vilib>:"Space Constant.vi"() -> ("String"=w146:string)
        n54 = call <vilib>:"Space Constant.vi"() -> ("String"=w145:string)
        n55 = call <vilib>:"Space Constant.vi"() -> ("String"=w143:string)
        n56 = Concatenate Strings("cd /home/pi/leakad", "\n", "sudo ./pipedaq ", "通道号", w147, "采样点数", w146, "采样率", w145, "增益", w143, "开始日期", w142, "开始时间", w141, "重复次数", w140, "时间间隔") -> (w139:string)
        n57 = call "Read Stream.vi"("Timout (s)"=10, "error in (no error)"=w161, "Connection Name"=w159, "Expected Response"="Expected Response", "Output ref"=w157) -> ("error out"=w167:errorcluster)  [unwired: 6 in]
        n58 = call "Is Connected.vi"("error in (no error)"=w167, "Connection Name"=w159) -> ("error out"=w166:errorcluster, "isSshConnected"=w152:bool)  [unwired: 8 in]
        n59 = call "计算采集时间.vi"("开始时间"="开始时间", "开始日期"="开始日期", "时间间隔"="时间间隔", "重复次数"="重复次数", "采样率"="采样率", "采样点数"="采样点数") -> ("时间延迟"=w128:i32, "采集时间"=w129:dbl)  [unwired: 4 in]
        n60 = call "Write.vi"("error in (no error)"=w166, "Connection Name"=w159, "Command"=w139) -> ("error out"=w130:errorcluster, "Return String"=w154:string)  [unwired: 7 in]
        n61 = call "Time Delay2"("error in (no error)"=w130, "Delay Time (s)"=w128) -> ("error out"=w127:errorcluster)  [unwired: 9 in]
        n62 = control-ref of="Output"() -> (w156:refnum<vi>)
        n63 = local write "isSshConnected"(w152) -> ()
        n64 = while {
          tunnel: w129 -> [w173]
          tunnel: w128 -> [w171]
          stop <- w174 stop-if-true
          # "进度条"
          n65 = property on="开始时间" class="DigNum (严格)"() -> ("Value"=w177:dbl)  [unwired: 2 in, 2 out]
          n66 = call <vilib>:"High Resolution Relative Seconds.vi"() -> ("relative seconds"=w178:dbl)
          n67 = Compound Arithmetic op=unknown(w171, w173, 14.0 ("值")) -> (w179:dbl)
          n68 = Subtract(x=w178, y=w177) -> (x-y=w172:dbl)
          n69 = Divide(x=w172, y=w179) -> (x/y=w176:dbl)
          "进度条" <- w176
          n70 = Greater Or Equal?(x=w176, y=1.0) -> (x >= y?=w174:bool)
        }
        n71 = local write "SSH响应"(w154) -> ()
        n72 = call "Read Stream.vi"("Timout (s)"=w129, "error in (no error)"=w127, "Connection Name"=w159, "Expected Response"="Expected Response", "Output ref"=w156) -> ("error out"=w164:errorcluster)  [unwired: 6 in]
        n73 = call "Time Delay"("error in (no error)"=w164, "Delay Time (s)"=2.0) -> ("error out"=w163:errorcluster)  [unwired: 9 in]
        n74 = call "Disconnect.vi"("error in (no error)"=w163, "Connection Name"=w159) -> ("error out"=w138:errorcluster, "isSshConnected"=w153:bool, "Return String"=w155:string)  [unwired: 7 in]
        n75 = local write "SSH响应"(w155) -> ()
        n76 = local write "isSshConnected"(w153) -> ()
        n77 = call <vilib>:"Add State(s) to Queue__JKI_lib_State_Machine.vi"("State(s) in (\"\")"=w170) -> ("States Out"=w169:string)  [unwired: 14 in]
      }
      frame "Alarm and Location" {
        w196 = "RF_analysis"  # function name
        # "调用Python节点，运行去噪和互相关算法，得到是否泄漏和泄漏位置"
        # "5"
        # "4"
        # "2"
        # "1"
        n78 = property on="采样率" class="Str"() -> ("Value"=w182:string)  [unwired: 2 in, 2 out]
        n79 = case shown="\"6\", 默认" w182 {
          tunnel: [1000 500 100 60 50 30] -> w181
          frame "5" {
          }
          frame "6", Default {
          }
          frame "7" {
          }
          frame "8" {
          }
          frame "9" {
          }
          frame "10" {
          }
        }
        n80 = property on="采样点数" class="Str"() -> ("Value"=w188:string)  [unwired: 2 in, 2 out]
        n81 = Decimal String To Number(string=w188) -> (number=w187:i32)  [unwired: 2 in, 1 out]
        n82 = call <vilib>:"Application Directory.vi"() -> ("Application Directory"=w201:path)
        n83 = call "ToPythonVersionString.vi"("Python版本"=PythonVersionsEnum."3.6") -> ("python版本字符串"=w199:string)  [unwired: 10 in]
        n84 = Build Path(base path=w201, name or relative path="References\\RF.py" ("名称或相对路径")) -> (appended path=w185:path)
        n85 = Open Python Session(python version=w199, 3:w203) -> (session out=w198:refnum<k35>, error out=w197:errorcluster)  [unwired: 1 in]
        n86 = node(w198, w185, w196, w197, cluster{bool, sgl} {TRUE, 0.0}, w187, w181, "管长") -> (w195:refnum<k35>, w194:errorcluster, w190:cluster{bool, sgl})  [unwired: 3 in, 2 out]
        n87 = Close Python Session(session in=w195, error in=w194) -> (11:w202:errorcluster)
        n88 = Unbundle(w190) -> (w183:bool, w186:sgl)
        "泄漏点位置" <- w186
        n89 = Number To Fractional String(number=w186, width (-)=i16 4 ("宽度(-)"), precision (6)=i16 2 ("精度(6)")) -> ()  [unwired: 1 in, 1 out]
        n90 = property on="运行状态" class="Bool (严格)"("Value"=w183) -> ()  [unwired: 2 in, 2 out]
        n91 = case shown="真" w183 {
          frame False {
            n92 = property on="诊断结论" class="Str"("Value"="运行状态良好！" ("诊断结论")) -> ()  [unwired: 2 in, 2 out]
          }
          frame True {
            n93 = property on="诊断结论" class="Str"("Value"="管道发生泄漏，请立即前往处理！" ("诊断结论")) -> ()  [unwired: 2 in, 2 out]
          }
        }
        n94 = call <vilib>:"Add State(s) to Queue__JKI_lib_State_Machine.vi"("State(s) in (\"\")"=w206) -> ("States Out"=w205:string)  [unwired: 14 in]
      }
      frame "Exit" {
        # "退出程序"
        # "Do not put any code in this frame.\n(No errors that occur here will be handled.)"
        n95 = call <vilib>:"Add State(s) to Queue__JKI_lib_State_Machine.vi"("State(s) in (\"\")"=w219) -> ("States Out"=w218:string)  [unwired: 14 in]
      }
      frame "---------- Data ----------" {
        # "Do not put any code in this frame.\n(It is a separator no-op. You can make a copy of this frame to create a new Data frame)"
        n96 = call <vilib>:"Add State(s) to Queue__JKI_lib_State_Machine.vi"("State(s) in (\"\")"=w223) -> ("States Out"=w222:string)  [unwired: 14 in]
      }
      frame "Data: Initialize" {
        w224 = T9 {"Current VI Reference"=refnum, "Close Panel on Exit?"=FALSE}  # Core
        w226 = TRUE  # Your Boolean data
        w225 = ""  # Your string data
        # "初始化移位寄存器"
        # "Expand Bundle to add new data elements to shift register data."
        # "Add new data here."
        # "Data names and types of shift register data are defined by this bundle."
        n97 = Bundle("Core"=w224, "Your Boolean data"=w226, "Your string data"=w225) -> (w228:T8)  [unwired: 1 in]
        n98 = call <vilib>:"Add State(s) to Queue__JKI_lib_State_Machine.vi"("State(s) in (\"\")"=w230) -> ("States Out"=w229:string)  [unwired: 14 in]
      }
      frame "Data: Transfer" {
        w232 = "Test Connection" ("Connection Name")
        w252 = 30  # Keep Alive Interval (s)
        # "SFTP读取数据文件"
        # "读取数据文件"
        # "读取log文件"
        n99 = case shown="\"第一台设备\", 默认" w246 {
          tunnel: [w263 w266 w269] -> w245
          tunnel: [w262 w265 w268] -> w244
          tunnel: ["Data\\1" ("字符串") "Data\\2" ("字符串") "Data\\3" ("字符串")] -> w243
          frame "第一台设备", Default {
            n100 = property on="Password 1" class="Clust (严格)"() -> ("Value"=w262:T3)  [unwired: 2 in, 2 out]
            n101 = property on="1号设备连接信息" class="Clust (严格)"() -> ("Value"=w263:T2)  [unwired: 2 in, 2 out]
          }
          frame "第二台设备" {
            n102 = property on="2号设备连接信息" class="Clust (严格)"() -> ("Value"=w266:T2)  [unwired: 2 in, 2 out]
            n103 = property on="Password 2" class="Clust (严格)"() -> ("Value"=w265:T3)  [unwired: 2 in, 2 out]
          }
          frame "第三台设备" {
            n104 = property on="3号设备连接信息" class="Clust (严格)"() -> ("Value"=w269:T2)  [unwired: 2 in, 2 out]
            n105 = property on="Password 3" class="Clust (严格)"() -> ("Value"=w268:T3)  [unwired: 2 in, 2 out]
          }
        }
        n106 = property on="Connection Type" class="Enum (严格)"() -> ("Value"=w249:enum16{"Password", "Private Key"})  [unwired: 2 in, 2 out]
        n107 = case shown="\"Private Key\"" w249 {
          tunnel: [w276 w281] -> w253
          tunnel: [w275 w280] -> _
          tunnel: [w274 w279] -> _
          tunnel: w250 -> [w273 w282]
          tunnel: w232 -> [w272 w278]
          tunnel: w245 -> [w271 w277]
          tunnel: w244 -> [w270 _]
          frame "Password", Default {
            n108 = call-poly "Connect.vi"("error in (no error)"=w273, "Connection Name"=w272, "Password"=w270, "Connection Info."=w271) -> ("error out"=w276:errorcluster, "isSftpConnected"=w275:bool, "Return String"=w274:string)  [unwired: 5 in]
          }
          frame "Private Key" {
            n109 = call-poly "Connect.vi"("error in (no error)"=w282, "Connection Name"=w278, "Connection Info."=w277) -> ("error out"=w281:errorcluster, "isSshConnected"=w280:bool, "Return String"=w279:string)  [unwired: 6 in]
          }
        }
        n110 = call "Keep Alive Interval.vi"("error in (no error)"=w253, "Connection Name"=w232, "Keep Alive Interval (s)"=w252) -> ("error out"=w254:errorcluster)  [unwired: 8 in]
        n111 = call <vilib>:"Application Directory.vi"() -> ("Application Directory"=w247:path)
        n112 = call "Is Connected.vi"("error in (no error)"=w254, "Connection Name"=w232) -> ("error out"=w236:errorcluster, "isSshConnected"=w257:bool)  [unwired: 8 in]
        n113 = local write "isSftpConnected"(w257) -> ()
        n114 = Build Path(base path=w247, name or relative path=w243) -> (appended path=w248:path)
        n115 = Empty String/Path?(string/path=w248) -> (empty?=w251:bool)
        n116 = case shown="真" w251 {
          tunnel: [w283 w284] -> w235
          tunnel: w248 -> [w283 _]
          frame False {
          }
          frame True {
            n117 = call "File Dialog"() -> ("selected path"=w284:path)  [unwired: 12 in, 3 out]
          }
        }
        n118 = call "Download File.vi"("error in (no error)"=w236, "Connection Name"=w232, "Local File Path"=w235, "Remote File Path"="/home/pi/leakad/log.dat") -> ("error out"=w231:errorcluster, "Return String"=w237:string)  [unwired: 6 in]
        n119 = local write "SFTP响应"(w237) -> ()
        n120 = call "读取数据文件.vi"("错误输入"=w231, "文件地址输入"=w235) -> ("错误输出"=w238:errorcluster, "Return String"=w233:string)  [unwired: 7 in, 1 out]
        n121 = local write "SFTP响应"(w233) -> ()
        n122 = call "时间延迟"("error in (no error)"=w238) -> ("error out"=w239:errorcluster)  [unwired: 10 in]
        n123 = call "Disconnect.vi"("error in (no error)"=w239, "Connection Name"=w232) -> ("error out"=w241:errorcluster, "isSshConnected"=w255:bool, "Return String"=w256:string)  [unwired: 7 in]
        n124 = local write "isSftpConnected"(w255) -> ()
        n125 = local write "SFTP响应"(w256) -> ()
        n126 = call "Time Delay3"("error in (no error)"=w241, "Delay Time (s)"=2.0) -> ("error out"=w240:errorcluster)  [unwired: 9 in]
        n127 = call <vilib>:"Add State(s) to Queue__JKI_lib_State_Machine.vi"("State(s) in (\"\")"=w260) -> ("States Out"=w259:string)  [unwired: 14 in]
      }
      frame "Data: Cleanup" {
        # "数据清理"
        n128 = Unbundle By Name(w285) -> ("Core.Current VI Reference"=w288:refnum<vi>)
        n129 = Close Reference(reference=w288, error in (no error)=w287) -> (error out=w286:errorcluster)
        n130 = call <vilib>:"Add State(s) to Queue__JKI_lib_State_Machine.vi"("State(s) in (\"\")"=w290) -> ("States Out"=w289:string)  [unwired: 14 in]
      }
      frame "---------- UI ----------" {
        # "UI界面分界线"
        n131 = call <vilib>:"Add State(s) to Queue__JKI_lib_State_Machine.vi"("State(s) in (\"\")"=w294) -> ("States Out"=w293:string)  [unwired: 14 in]
      }
      frame "UI: Initialize" {
        # "初始化用户界面"
        n132 = property on="进度条" class="Slide (严格)"("Value"=0.0 ("进度条")) -> ()  [unwired: 2 in, 2 out]
        n133 = call "自适应屏幕分辨率.vi"("error in (no error)"=w295) -> ("error out"=w296:errorcluster)
        n134 = call <vilib>:"Add State(s) to Queue__JKI_lib_State_Machine.vi"("State(s) in (\"\")"=w300) -> ("States Out"=w299:string)  [unwired: 14 in]
      }
      frame "UI: Display" {
        n135 = call <vilib>:"Application Directory.vi"() -> ("Application Directory"=w319:path)
        n136 = call <vilib>:"Application Directory.vi"() -> ("Application Directory"=w307:path)
        n137 = call <vilib>:"Application Directory.vi"() -> ("Application Directory"=w313:path)
        n138 = Build Path(base path=w319, name or relative path="Data\\1\\log.dat" ("名称或相对路径")) -> (appended path=w317:path)
        n139 = Build Path(base path=w307, name or relative path="Data\\3\\log.dat" ("名称或相对路径")) -> (appended path=w305:path)
        n140 = Build Path(base path=w313, name or relative path="Data\\2\\log.dat" ("名称或相对路径")) -> (appended path=w315:path)
        n141 = Read from Text File(file (use dialog)=w317) -> (text=w321:string)  [unwired: 3 in, 3 out]
        n142 = Read from Text File(file (use dialog)=w305) -> (text=w309:string)  [unwired: 3 in, 3 out]
        n143 = Read from Text File(file (use dialog)=w315) -> (text=w311:string)  [unwired: 3 in, 3 out]
        n144 = String Subset(string=w321, offset (0)=2 ("偏移量(0)"), length (rest)=22 ("长度（剩余）")) -> (substring=w316:string)
        n145 = String Subset(string=w309, offset (0)=2 ("偏移量(0)"), length (rest)=22 ("长度（剩余）")) -> (substring=w304:string)
        n146 = String Subset(string=w311, offset (0)=2 ("偏移量(0)"), length (rest)=22 ("长度（剩余）")) -> (substring=w310:string)
        n147 = call <vilib>:"Application Directory.vi"() -> ("Application Directory"=w335:path)
        n148 = Concatenate Strings("Data\\2\\" ("名称或相对路径"), w310) -> (w325:string)
        n149 = call <vilib>:"Application Directory.vi"() -> ("Application Directory"=w336:path)
        n150 = Concatenate Strings("Data\\3\\" ("名称或相对路径"), w304) -> (w322:string)
        n151 = Concatenate Strings("Data\\1\\" ("名称或相对路径"), w316) -> (w326:string)
        n152 = call <vilib>:"Application Directory.vi"() -> ("Application Directory"=w338:path)
        n153 = Build Path(base path=w335, name or relative path=w325) -> (appended path=w334:path)
        n154 = Build Path(base path=w336, name or relative path=w322) -> (appended path=w333:path)
        n155 = Build Path(base path=w338, name or relative path=w326) -> (appended path=w337:path)
        n156 = call-poly <vilib>:"Read Delimited Spreadsheet.vi"("file path (dialog if empty)"=w337, "transpose? (F)"=TRUE) -> ("first row"=w332:dbl[])  [unwired: 8 in, 5 out]
        n157 = call-poly <vilib>:"Read Delimited Spreadsheet.vi"("file path (dialog if empty)"=w334, "transpose? (F)"=TRUE) -> ("first row"=w331:dbl[])  [unwired: 8 in, 5 out]
        n158 = call-poly <vilib>:"Read Delimited Spreadsheet.vi"("file path (dialog if empty)"=w333, "transpose? (F)"=TRUE) -> ("first row"=w330:dbl[])  [unwired: 8 in, 5 out]
        n159 = Bundle("first row"=w332, "first row"=w331, "first row"=w330) -> (→"混合信号图":T1)  [unwired: 1 in]
        n160 = property on="混合信号图" class="MixedGraph (严格)"("Plot Area Colors"=T7 {"Foreground Color"=0, "Background Color"=16448250} ("绘图区域:颜色")) -> ()  [unwired: 2 in, 2 out]
        n161 = Wait Until Next ms Multiple(millisecond multiple=u32 100 ("毫秒倍数")) -> ()  [unwired: 1 out]
        n162 = call <vilib>:"Add State(s) to Queue__JKI_lib_State_Machine.vi"("State(s) in (\"\")"=w346) -> ("States Out"=w345:string)  [unwired: 14 in]
      }
      frame "UI: Cursor Set" {
        # "Argument"
        # "设置光标忙碌或者闲置\n(Usage: \"UI: Cursor Set >> Busy|Idle\")"
        n163 = case shown="\"Busy\"" w347 {
          tunnel: w349 -> [w354 w356]
          tunnel: [w353 w355] -> w348
          frame "Idle", Default {
            n164 = call <vilib>:"Unset Busy.vi"("error in (no error)"=w354) -> ("error out"=w353:errorcluster)  [unwired: 10 in]
          }
          frame "Busy" {
            n165 = call <vilib>:"Set Busy.vi"("error in (no error)"=w356) -> ("error out"=w355:errorcluster)  [unwired: 9 in, 1 out]
          }
        }
        n166 = call <vilib>:"Add State(s) to Queue__JKI_lib_State_Machine.vi"("State(s) in (\"\")"=w352) -> ("States Out"=w351:string)  [unwired: 14 in]
      }
      frame "UI: Front Panel State" {
        # "Argument"
        # "设置前面板开关\n(Usage: \"UI: Front Panel State >> Open|Close\")"
        n167 = Unbundle By Name(w359) -> ("Core.Current VI Reference"=w358:refnum<vi>)
        n168 = case shown="\"Maximize\", \"Maximized\"" w357 {
          tunnel: w361 -> [w369 w384 w395 w408 w421]
          tunnel: [w371 w385 w397 w410 w423] -> w360
          tunnel: w358 -> [w370 w382 w396 w409 w422]
          frame "Open", "Standard", Default {
            w364 = T4."Standard" ("State")
            n169 = property class="VI"(reference=w370, error in=w369) -> (reference out=w367:refnum<vi>, error out=w368:errorcluster, "FP.State"=w366:T4)
            n170 = Not Equal?(x=w366, y=w364) -> (x != y?=w365:bool)
            n171 = case shown="真" w365 {
              tunnel: [w375 w377] -> w371
              tunnel: w368 -> [w374 w377]
              tunnel: w367 -> [w373 _]
              tunnel: w364 -> [w372 _]
              frame True {
                n172 = invoke class="VI" method="FP.Open"(reference=w373, error in=w374, "Activate"=TRUE, "State"=w372) -> (error out=w375:errorcluster)  [unwired: 1 in, 4 out]
              }
              frame False {
              }
            }
          }
          frame "Close", "Closed" {
            n173 = property class="VI"(reference=w382, error in=w384) -> (reference out=w381:refnum<vi>, error out=w383:errorcluster, "FP.State"=w379:T4)
            n174 = Not Equal?(x=w379, y=T4."Closed" ("Front Panel Window:State")) -> (x != y?=w378:bool)
            n175 = case shown="真" w378 {
              tunnel: [w386 w389] -> w385
              tunnel: w383 -> [w386 w388]
              tunnel: w381 -> [_ w387]
              frame False {
              }
              frame True {
                n176 = invoke class="VI" method="FP.Close"(reference=w387, error in=w388) -> (error out=w389:errorcluster)  [unwired: 1 in, 2 out]
              }
            }
          }
          frame "Hidden", "Hide" {
            w390 = T4."Hidden" ("State")
            n177 = property class="VI"(reference=w396, error in=w395) -> (reference out=w393:refnum<vi>, error out=w394:errorcluster, "FP.State"=w392:T4)
            n178 = Not Equal?(x=w392, y=w390) -> (x != y?=w391:bool)
            n179 = case shown="真" w391 {
              tunnel: [w401 w402] -> w397
              tunnel: w394 -> [w400 w402]
              tunnel: w393 -> [w399 _]
              tunnel: w390 -> [w398 _]
              frame True {
                n180 = invoke class="VI" method="FP.Open"(reference=w399, error in=w400, "State"=w398) -> (error out=w401:errorcluster)  [unwired: 2 in, 4 out]
              }
              frame False {
              }
            }
          }
          frame "Minimize", "Minimized" {
            w403 = T4."Minimized" ("State")
            n181 = property class="VI"(reference=w409, error in=w408) -> (reference out=w406:refnum<vi>, error out=w407:errorcluster, "FP.State"=w405:T4)
            n182 = Not Equal?(x=w405, y=w403) -> (x != y?=w404:bool)
            n183 = case shown="真" w404 {
              tunnel: [w414 w415] -> w410
              tunnel: w407 -> [w413 w415]
              tunnel: w406 -> [w412 _]
              tunnel: w403 -> [w411 _]
              frame True {
                n184 = invoke class="VI" method="FP.Open"(reference=w412, error in=w413, "State"=w411) -> (error out=w414:errorcluster)  [unwired: 2 in, 4 out]
              }
              frame False {
              }
            }
          }
          frame "Maximize", "Maximized" {
            w416 = T4."Maximized" ("State")
            n185 = property class="VI"(reference=w422, error in=w421) -> (reference out=w419:refnum<vi>, error out=w420:errorcluster, "FP.State"=w418:T4)
            n186 = Not Equal?(x=w418, y=w416) -> (x != y?=w417:bool)
            n187 = case shown="真" w417 {
              tunnel: [w427 w428] -> w423
              tunnel: w420 -> [w426 w428]
              tunnel: w419 -> [w425 _]
              tunnel: w416 -> [w424 _]
              frame True {
                n188 = invoke class="VI" method="FP.Open"(reference=w425, error in=w426, "State"=w424) -> (error out=w427:errorcluster)  [unwired: 2 in, 4 out]
              }
              frame False {
              }
            }
          }
        }
        n189 = call <vilib>:"Add State(s) to Queue__JKI_lib_State_Machine.vi"("State(s) in (\"\")"=w363) -> ("States Out"=w362:string)  [unwired: 14 in]
      }
      frame "---------- Macro ----------" {
        # "Do not put any code in this frame.\n(It is a separator no-op. You can make a copy of this frame to create a new Macro frame)"
        n190 = call <vilib>:"Add State(s) to Queue__JKI_lib_State_Machine.vi"("State(s) in (\"\")"=w432) -> ("States Out"=w431:string)  [unwired: 14 in]
      }
      frame "Macro: Initialize" {
        # "跳转到初始化事件"
        # "宏指令"
        n191 = call <vilib>:"Add State(s) to Queue__JKI_lib_State_Machine.vi"("State(s) in Front (\"\")"="Data: Initialize\nInitialize Core Data\nUI: Initialize\nUI: Front Panel State >> Maximize", "State(s) in (\"\")"=w437) -> ("States Out"=w436:string)  [unwired: 13 in]
      }
      frame "Macro: Run" {
        w438 = "Device Connected>>第一台设备\nAcquire Data\nData: Transfer>>第一台设备\n//Device Connected>>第二台设备\n//Acquire Data\n//Data: Transfer>>第二台设备\n//Device Connected>>第三台设备\n//Acquire Data\n//Data: Transfer>>第三台设备\nUI: Display\nAlarm and Location"  # Device Connected>>第一台设备 Acquire Data Data: Transfer>>第一台设备 //Device Connected>>第二台设备 //Acquire Data //Data: Transfer>>第二台设备 //Device Connected>>第三台设备 //Acquire Data //Data: Transfer>>第三台设备 UI: Display Alarm and Location
        n192 = call <vilib>:"Add State(s) to Queue__JKI_lib_State_Machine.vi"("State(s) in Front (\"\")"=w438, "State(s) in (\"\")"=w442) -> ("States Out"=w441:string)  [unwired: 13 in]
      }
      frame "Macro: Exit" {
        # "宏指令：退出程序"
        n193 = Unbundle By Name(w449) -> ("Core.Close Panel on Exit?"=w448:bool)
        n194 = Select(t="UI: Front Panel State >> Close", s=w448, f="") -> (s? t:f=w445:string)
        n195 = call <vilib>:"Add State(s) to Queue__JKI_lib_State_Machine.vi"("State(s) in (\"\")"=w445, "State(s) at Back (\"\")"="Data: Cleanup\nExit") -> ("States Out"=w443:string)  [unwired: 13 in]
        n196 = call <vilib>:"Add State(s) to Queue__JKI_lib_State_Machine.vi"("State(s) in Front (\"\")"=w443, "State(s) in (\"\")"=w452) -> ("States Out"=w451:string)  [unwired: 13 in]
      }
    }
  }
